vi "Create Incrementing Suffix File Path.vi"(7 "format string (\" (%d)\")":string=" (%d)", 8 "error in":errorcluster, 11 "file path":path) -> (0 "error out":errorcluster, 3 "actual path":path)   [LabVIEW 2020]
doc: "Works in similar way as the inbuilt LV function \"Create File with Incrementing Suffix\" but does not create the file reference. Instead it returns the new path, so it can be used with any file type e.g. txt, TDMS etc."
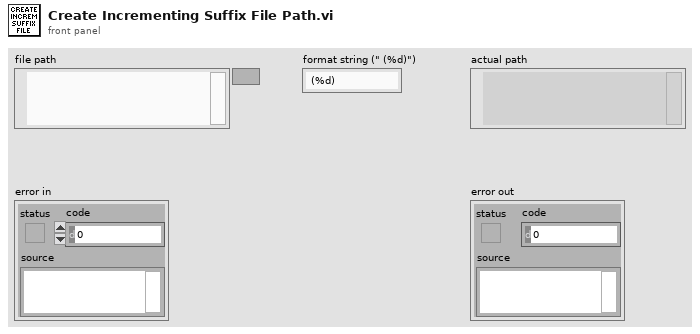
[diagram p1: front panel]
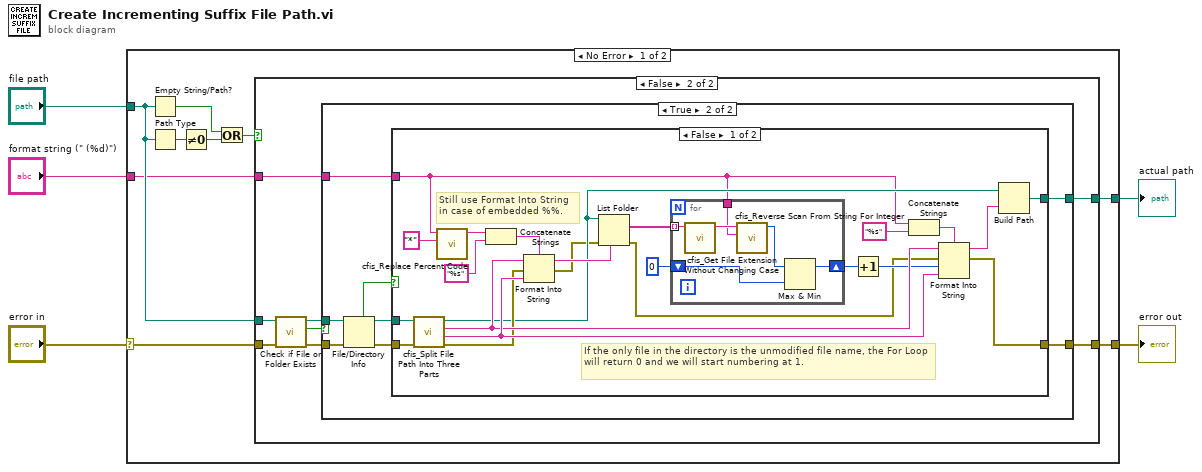
[diagram p0: block diagram]
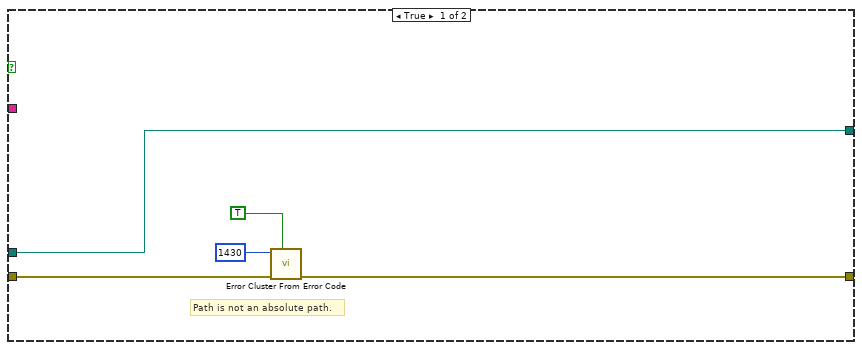
[diagram p2: hidden frame]
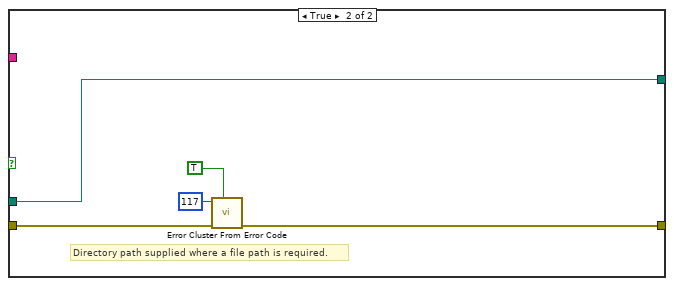
[diagram p4: hidden frame]
diagram:
  n1 = case shown="No Error" "error in" {
    selector: "error in" -> [w13 w72]
    tunnel: "file path" -> [w8 w71]
    tunnel: [w14 w72] -> w4
    tunnel: [w7 w71] -> w2
    tunnel: "format string (\" (%d)\")" -> [w6 _]
    frame No Error {
      n2 = Empty String/Path?(string/path=w8) -> (empty?=w10:bool)
      n3 = Path Type(1:w8) -> (0:w12:i16)
      n4 = Not Equal To 0?(x=w12) -> (x != 0?=w11:bool)
      n5 = Or(x=w10, y=w11) -> (x .or. y?=w9:bool)
      n6 = case shown="False" w9 {
        tunnel: [w19 w20] -> w14
        tunnel: w13 -> [w17 w27]
        tunnel: w8 -> [w15 w26]
        tunnel: [w15 w22] -> w7
        tunnel: w6 -> [_ w21]
        frame True {
          # "Path is not an absolute path."
          n7 = call <vilib>:"Error Cluster From Error Code.vi"("show call chain? (False)"=TRUE, "error in (no error)"=w17, "error code (0)"=1430) -> ("error out"=w19:errorcluster)  [unwired: 6 in]
        }
        frame False {
          n8 = call <vilib>:"Check if File or Folder Exists.vi"("error in (no error)"=w27, "path"=w26) -> ("error out"=w23:errorcluster, "file or folder exists?"=w25:bool, "dup path"=w24:path)  [unwired: 7 in]
          n9 = case shown="True" w25 {
            tunnel: w24 -> [w29 w37]
            tunnel: [w29 w31] -> w22
            tunnel: w23 -> [w28 w36]
            tunnel: [w28 w33] -> w20
            tunnel: w21 -> [_ w30]
            frame False {
            }
            frame True {
              n10 = File/Directory Info(path=w37, error in=w36) -> (path out=w32:path, directory=w35:bool, error out=w34:errorcluster)  [unwired: 4 out]
              n11 = case shown="False" w35 {
                tunnel: w34 -> [w50 w70]
                tunnel: [w40 w67] -> w33
                tunnel: w32 -> [w59 w66]
                tunnel: [w41 w66] -> w31
                tunnel: w30 -> [w38 _]
                frame False {
                  # "If the only file in the directory is the unmodified file name, the For Loop will return 0 and we will start numbering at 1."
                  # "Still use Format Into String\nin case of embedded %%."
                  n12 = call <vilib>:"cfis_Split File Path Into Three Parts.vi"("file path"=w59) -> ("File extension"=w52:string, "File name without extension"=w51:string, "Directory"=w48:path)  [unwired: 8 in]
                  n13 = call <vilib>:"cfis_Replace Percent Code.vi"("replace text"="*", "format string in"=w38) -> ("format string out"=w55:string)  [unwired: 9 in]
                  n14 = Concatenate Strings(w55, "%s" ("format string")) -> (w54:string)
                  n15 = Format Into String(format string=w54, initial string=w51, error in=w50, w52) -> (resulting string=w49:string, error out=w47:errorcluster)
                  n16 = List Folder(path=w48, pattern=w49, error in=w47) -> (filenames=w46:string[], error out=w39:errorcluster)  [unwired: 1 in, 2 out]
                  n17 = for {
                    tunnel: w46 -> [w65] mode=indexing
                    shift-right: [w61] -> w44
                    shift-left: 0 -> [w62]
                    tunnel: w38 -> [w60]
                    n18 = call <vilib>:"cfis_Get File Extension Without Changing Case.vi"("file name"=w65) -> ("file name without extension"=w64:string)  [unwired: 9 in, 1 out]
                    n19 = call <vilib>:"cfis_Reverse Scan From String For Integer.vi"("format string"=w60, "input string"=w64) -> ("Extracted integer"=w63:i32)  [unwired: 9 in]
                    n20 = Max & Min(x=w63, y=w62) -> (max(x,y)=w61:i32)  [unwired: 1 out]
                  }
                  n21 = Increment(x=w44) -> (x+1=w42:i32)
                  n22 = Concatenate Strings(w38, "%s" ("format string")) -> (w57:string)
                  n23 = Format Into String(format string=w57, initial string=w51, error in=w39, w42, w52) -> (resulting string=w43:string, error out=w40:errorcluster)
                  n24 = Build Path(base path=w48, name or relative path=w43) -> (appended path=w41:path)
                }
                frame True {
                  # "Directory path supplied where a file path is required."
                  n25 = call <vilib>:"Error Cluster From Error Code.vi"("show call chain? (False)"=TRUE, "error in (no error)"=w70, "error code (0)"=117) -> ("error out"=w67:errorcluster)  [unwired: 6 in]
                }
              }
            }
          }
        }
      }
    }
    frame Error {
    }
  }
  "error out" <- w4
  "actual path" <- w2
